vi "ConfigureWindowsPowerManagement.vi"(8 "ErrorIn":errorcluster) -> (0 "ErrorOut":errorcluster)   [LabVIEW 2018]
doc: "This VI is used to set the Windows Power Management Options. This is often valuable when you have an application that will not respond well to Window shutting down, going to standby, dimming the screen, etc.\n\nCopyright © 2011 Epimedia, Inc. All Rights Reserved.\n\nThe Epimedia Application Library is Copyright © 2009-2011 Epimedia, Inc. \nAll Rights Reserved. Used under license."
panel:
  # "Copyright © 2011 Epimedia, Inc. All Rights Reserved.\n\nThe Epimedia Application Library is Copyright © 2009-2011 Epimedia, Inc. \nAll Rights Reserved. Used under license."
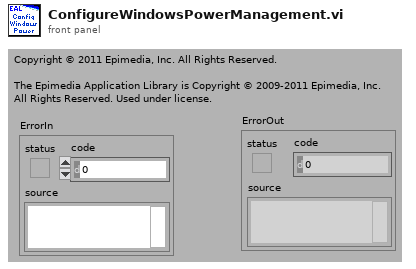
[diagram p1: front panel]
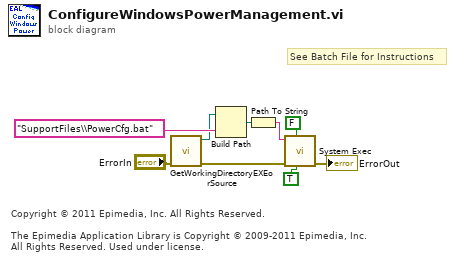
[diagram p0: block diagram]
diagram:
  # "Copyright © 2011 Epimedia, Inc. All Rights Reserved.\n\nThe Epimedia Application Library is Copyright © 2009-2011 Epimedia, Inc. \nAll Rights Reserved. Used under license."
  # "See Batch File for Instructions"
  n1 = call "GetWorkingDirectoryEXEorSource.vi"("ErrorIn"="ErrorIn") -> ("ErrorOut"=w1:errorcluster, "Directory"=w2:path)  [unwired: 9 in]
  n2 = Build Path(base path=w2, name or relative path="SupportFiles\\PowerCfg.bat") -> (appended path=w5:path)
  n3 = Path To String(path=w5) -> (string=w4:string)
  n4 = call <vilib>:"System Exec.vi"("run minimized? (F)"=TRUE ("wait until completion? (T)"), "wait until completion? (T)"=FALSE, "error in (no error)"=w1, "command line"=w4) -> ("error out"=→"ErrorOut":errorcluster)  [unwired: 2 in, 5 out]
